vi "Drag Panel-Set Parent Window.vi"(8 "error in":errorcluster, 10 "Parent Window ID":u32, 11 "Child Window ID":u32) -> (0 "error out":errorcluster, 3 "Return Type":u32)   [LabVIEW 2015]
uses:
  USER32.DLL
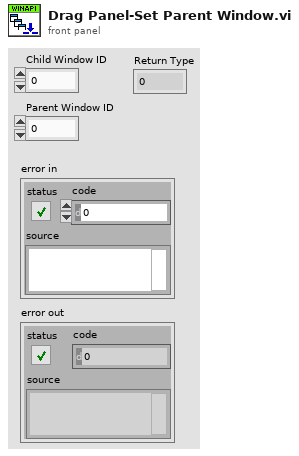
[diagram p1: front panel]
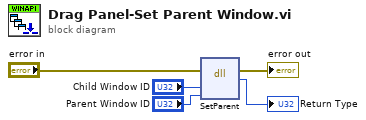
[diagram p0: block diagram]
diagram:
  n1 = dll-call lib="user32.dll" fn="SetParent"(error in="error in", "Child"="Child Window ID", "NewParent"="Parent Window ID") -> (error out=→"error out":errorcluster, "return type"=→"Return Type":u32)  [unwired: 4 in, 1 out]
